vi "ROS_Read_LIDAR.vi"(8 "error in (no error)":errorcluster, 11 "scan_in":T2={"topic port"=0, "Node"="", "topic"="", "type"="", "node port"=0, "error "={"status"=FALSE, "code"=0, "source"=""}, "Direction"=enum."Node", "Update (ms)"=1, "FIFO size"=1}) -> (0 "error out":errorcluster, 1 "new?":bool, 2 "LaserScan_msg":T1, 3 "scan_out":T2={"topic port"=0, "Node"="", "topic"="", "type"="", "node port"=0, "error "={"status"=FALSE, "code"=0, "source"=""}, "Direction"=enum."Node", "Update (ms)"=1, "FIFO size"=1})   [LabVIEW 2017]
doc: "Read LIDAR sensor data from ROS topic\nnew? is TRUE when the message read has a different sequence ID as the last one read by the VI"
uses:
  <vilib>/Tufts CEEO ROS for LabVIEW Software/ROS/Code/SubVIs/_ROSControl.ctl
  <vilib>/Tufts CEEO ROS for LabVIEW Software/ROS/Code/SubVIs/_ROSDirection.ctl
  LaserScan.ctl
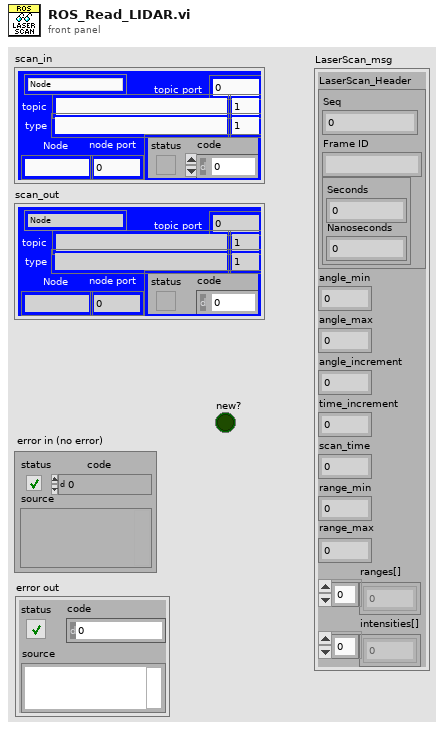
[diagram p1: front panel]
types:
  T1 = typedef "LaserScan.ctl" = cluster{"LaserScan_Header":cluster{"Seq":u32, "Frame ID":string, cluster{"Seconds":i32, "Nanoseconds":i32}}, "angle_min":dbl, "angle_max":dbl, "angle_increment":dbl, "time_increment":dbl, "scan_time":dbl, "range_min":dbl, "range_max":dbl, "ranges[]":dbl[], "intensities[]":dbl[]}
  T2 = typedef "_ROSControl.ctl" = cluster{"topic port":u16, "Node":string, "topic":string, "type":string, "node port":u16, "error ":errorcluster, "Direction":T3, "Update (ms)":u16, "FIFO size":u16}
  T3 = typedef "_ROSDirection.ctl" = enum16{"Node", "Publisher", "Subscriber", "ServiceClient", "ServiceProvider"}
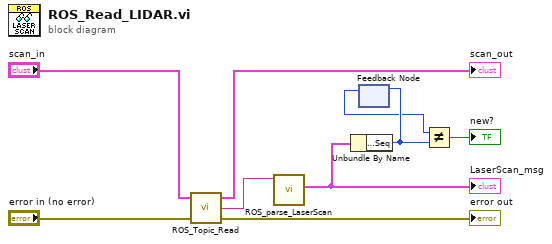
[diagram p0: block diagram]
diagram:
  n1 = call <vilib>:"ROS_Topic_Read.vi"("error in (no error)"="error in (no error)", "ROS in"="scan_in") -> ("error out"=→"error out":errorcluster, "Reply"=w5:string, "ROS out"=→"scan_out":T2)  [unwired: 1 in]
  n2 = call "ROS_parse_LaserScan.vi"("msg in"=w5) -> ("LaserScan_msg"=w4:T1)  [unwired: 9 in, 1 out]
  "LaserScan_msg" <- w4
  n3 = Unbundle By Name(w4) -> ("LaserScan_Header.Seq"=w3:u32)
  n4 = feedback-in #1(w3) -> ()
  n5 = feedback #1() -> (w2:u32)  [unwired: 1 in]
  n6 = Not Equal?(x=w2, y=w3) -> (x != y?=→"new?":bool)
